vi "solar_app Resolve Name.vi"(0 "Name to Resolve (\"\"=default Name)":string, 1 "default Name":string) -> (6 "Resolved Name":string)   [LabVIEW 2018]
doc: "This resolves a name by removing invalid characters. Allowed characters: [a-zA-Z0-9_]"
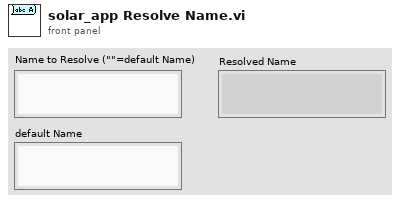
[diagram p1: front panel]
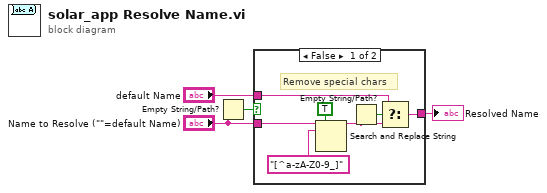
[diagram p0: block diagram]
diagram:
  n1 = Empty String/Path?(string/path="Name to Resolve (\"\"=default Name)") -> (empty?=w4:bool)
  n2 = case shown="False" w4 {
    tunnel: "Name to Resolve (\"\"=default Name)" -> [w8 _]
    tunnel: "default Name" -> [w6 w12]
    tunnel: [w7 w12] -> w1
    frame False {
      # "Remove special chars"
      n3 = Search and Replace String(replace all?=TRUE, input string=w8, search string="[^a-zA-Z0-9_]") -> (result string=w5:string)  [unwired: 5 in, 3 out]
      n4 = Empty String/Path?(string/path=w5) -> (empty?=w9:bool)
      n5 = Select(t=w6, s=w9, f=w5) -> (s? t:f=w7:string)
    }
    frame True {
    }
  }
  "Resolved Name" <- w1
